vi "Sub06_MatlabExecuter.vi"(8 "error in (no error)":errorcluster, 11 "String":string) -> (0 "error out":errorcluster, 2 "matlab standard error":string, 3 "matlab standard output":string)   [LabVIEW 2019]
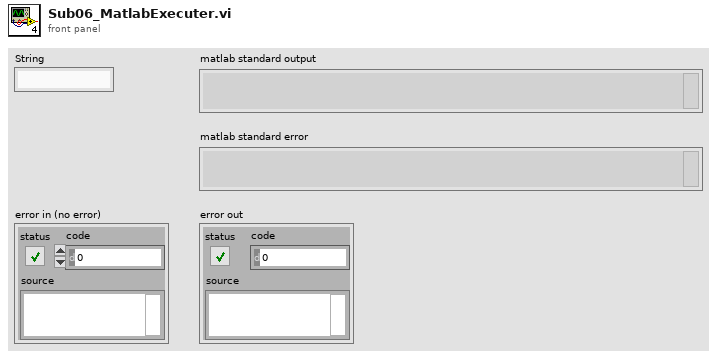
[diagram p1: front panel]
types:
  T1 = enum16{"open", "replace", "create", "open or create", "replace or create", "replace or create with confirmation"}
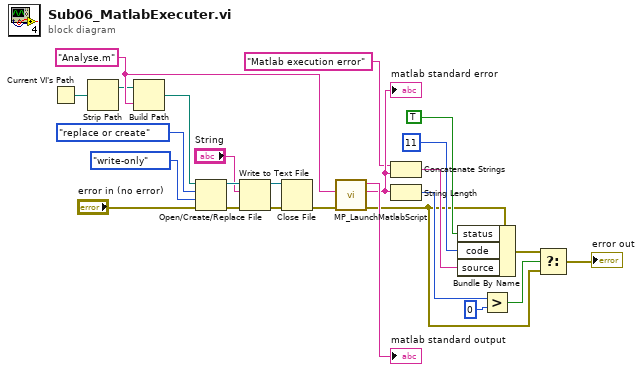
[diagram p0: block diagram]
diagram:
  w15 = "Analyse.m" ("File name in")
  n1 = Current VI's Path() -> (path=w9:path)
  n2 = Strip Path(path=w9) -> (stripped path=w8:path)  [unwired: 1 out]
  n3 = Build Path(base path=w8, name or relative path=w15) -> (appended path=w25:path)
  n4 = Open/Create/Replace File(file path (use dialog)=w25, error in="error in (no error)", operation (0:open)=T1."replace or create", access (0:read/write)=enum16{"read/write", "read-only", "write-only"}."write-only") -> (refnum out=w21:refnum<file>, error out=w24:errorcluster)  [unwired: 2 in, 1 out]
  n5 = Write to Text File(file (use dialog)=w21, text="String", error in=w24) -> (refnum out=w22:refnum<file>, error out=w23:errorcluster)  [unwired: 1 in, 1 out]
  n6 = Close File(refnum=w22, error in=w23) -> (error out=w16:errorcluster)  [unwired: 1 out]
  n7 = call "MP_LaunchMatlabScript.vi"("error in (no error)"=w16, "matlab script name with extension"=w15) -> ("error out"=w2:errorcluster, "standard error"=w7:string, "standard output"=→"matlab standard output":string)  [unwired: 5 in, 2 out]
  "matlab standard error" <- w7
  n8 = Concatenate Strings("Matlab execution error" ("string"), w7) -> (w5:string)
  n9 = String Length(string=w7) -> (length=w4:i32)
  n10 = Bundle By Name(cluster=w2, "status"=TRUE, "code"=11, "source"=w5) -> (w1:errorcluster)
  n11 = Greater?(x=w4, y=0) -> (0:w12:bool)
  n12 = Select(t=w1, s=w12, f=w2) -> (s? t:f=→"error out":errorcluster)
